vi "UHR-Fleezers Control (host) - 10.8.vi"() -> ()   [LabVIEW 2013] (continued)
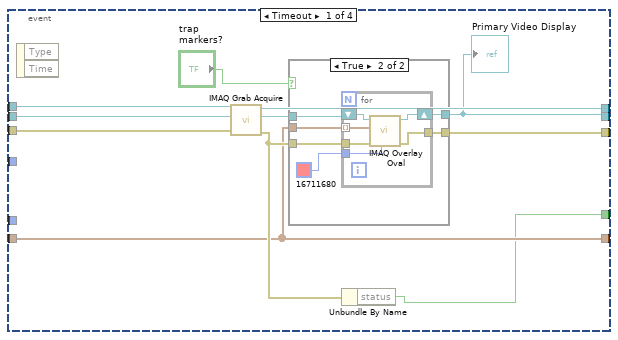
[diagram p2: hidden frame]
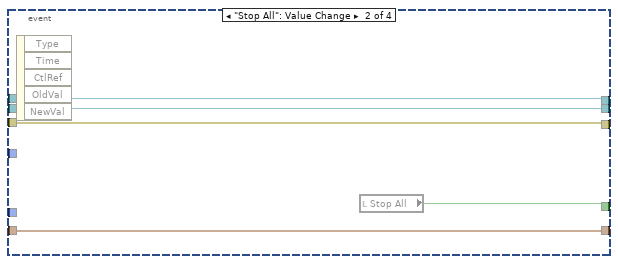
[diagram p4: hidden frame]
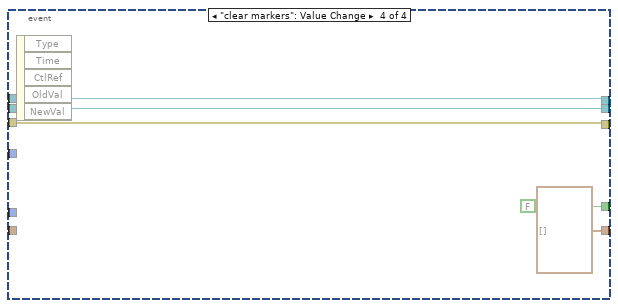
[diagram p6: hidden frame]
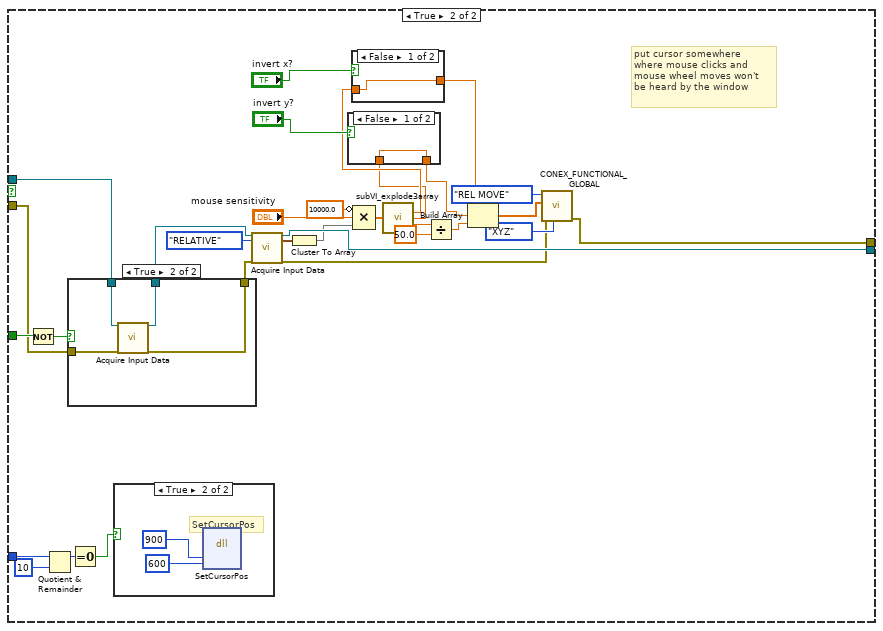
[diagram p9: hidden frame]
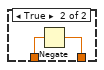
[diagram p12: hidden frame]
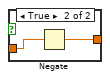
[diagram p13: hidden frame]
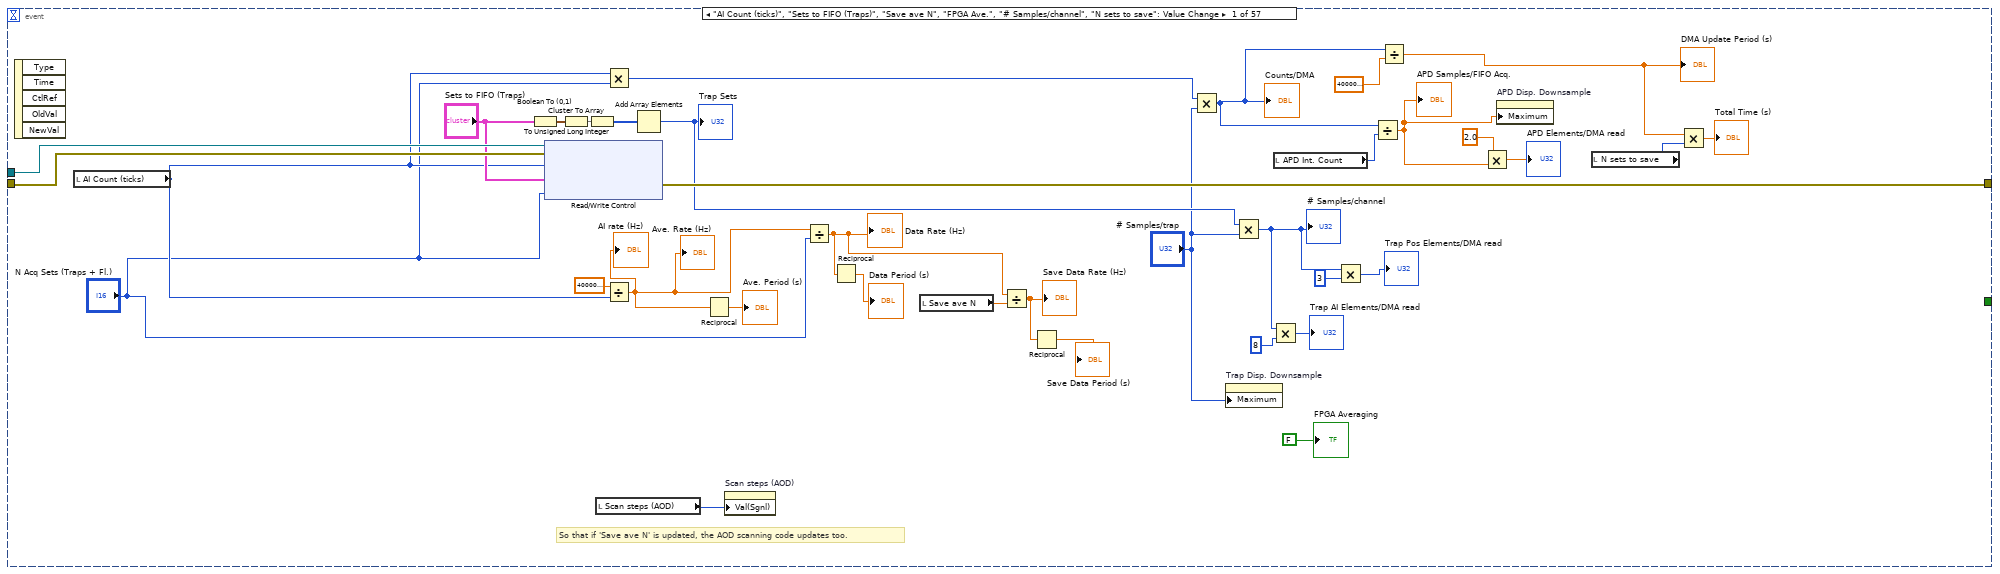
[diagram p14: hidden frame]
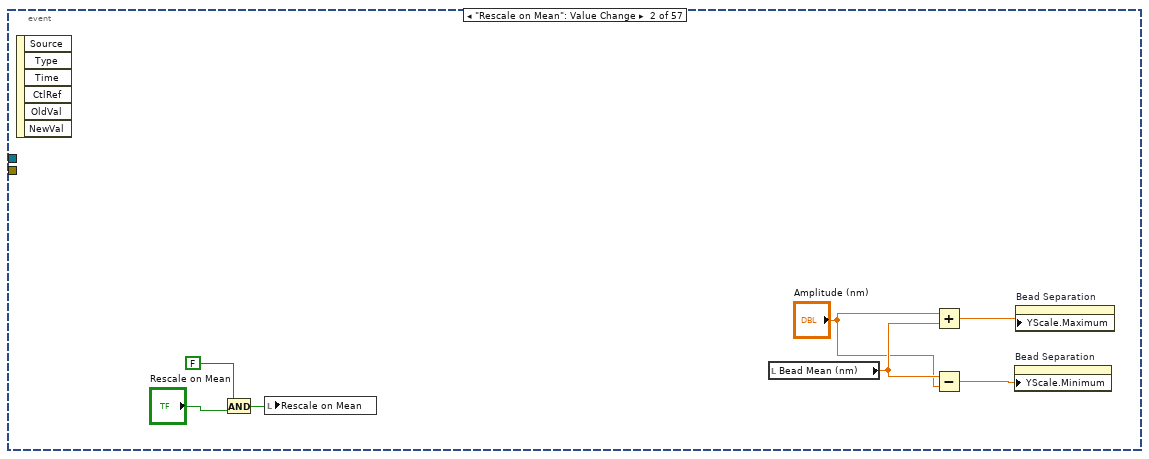
[diagram p15: hidden frame]
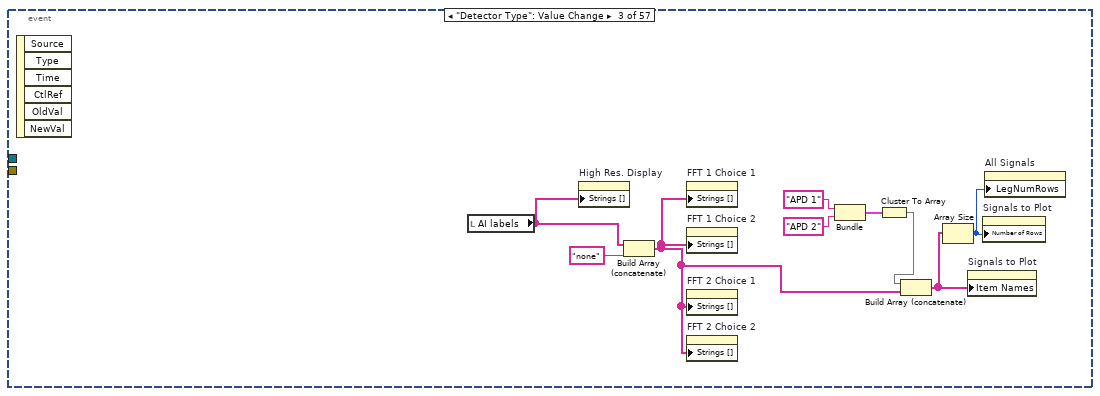
[diagram p16: hidden frame]
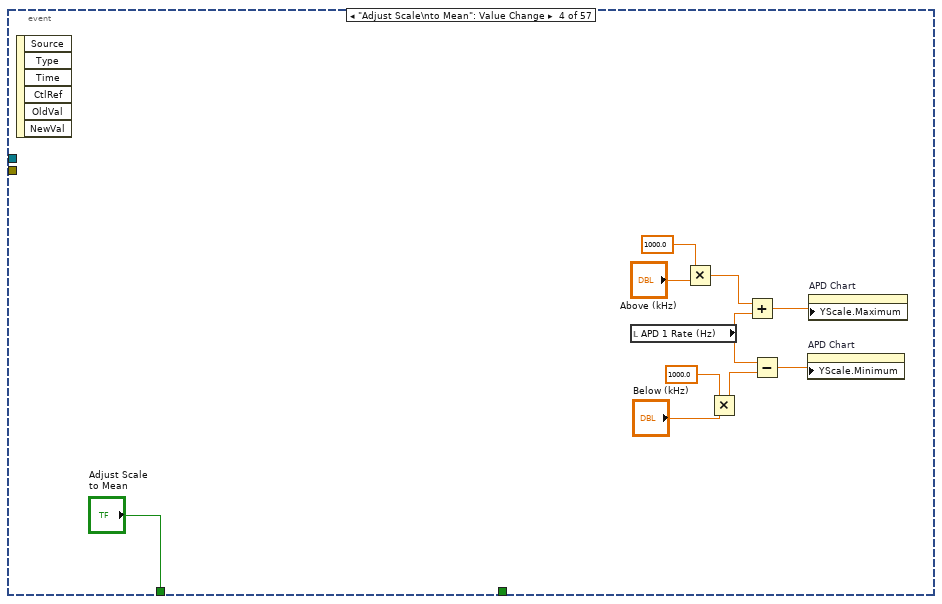
[diagram p17: hidden frame]
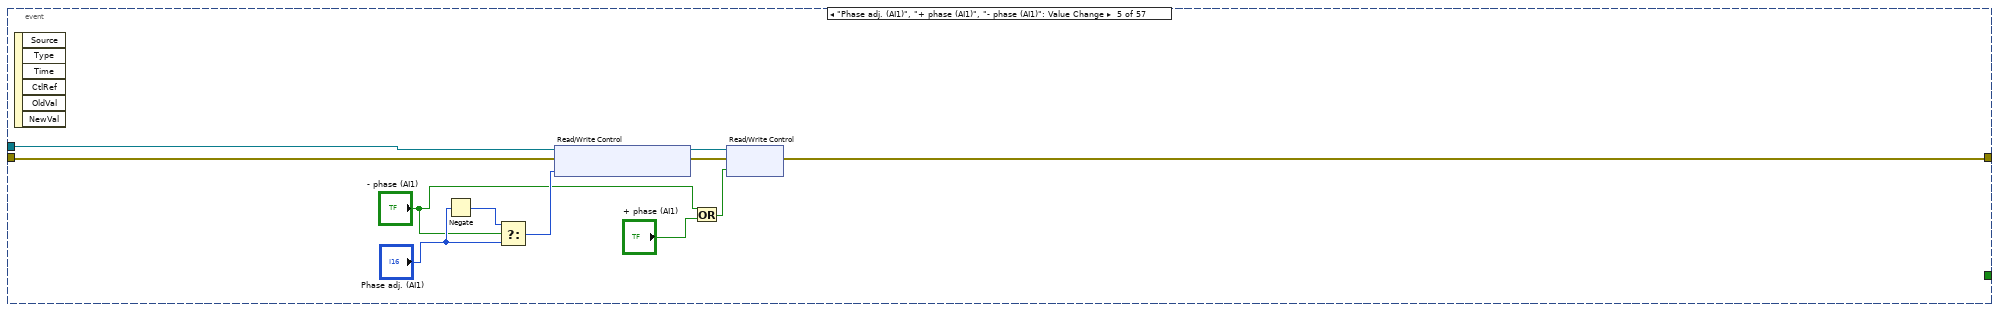
[diagram p18: hidden frame]
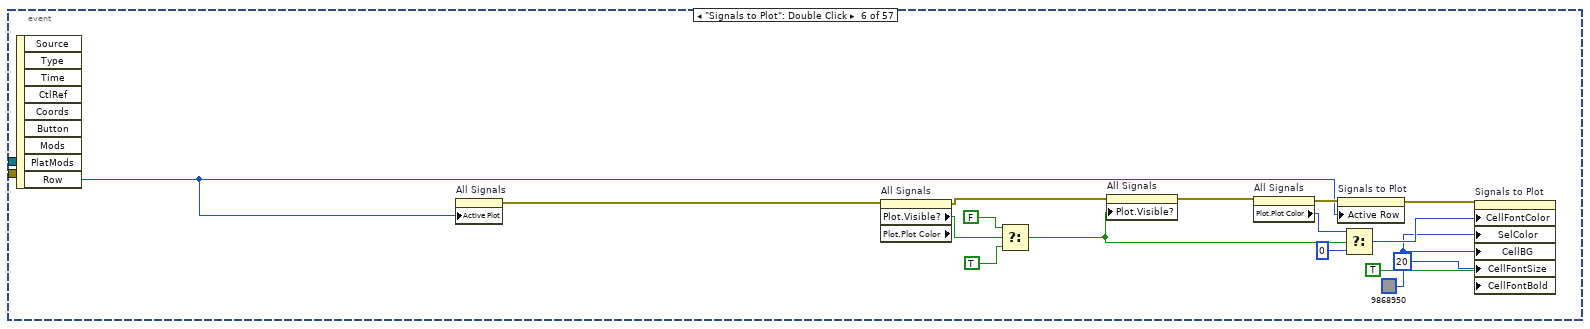
[diagram p19: hidden frame]
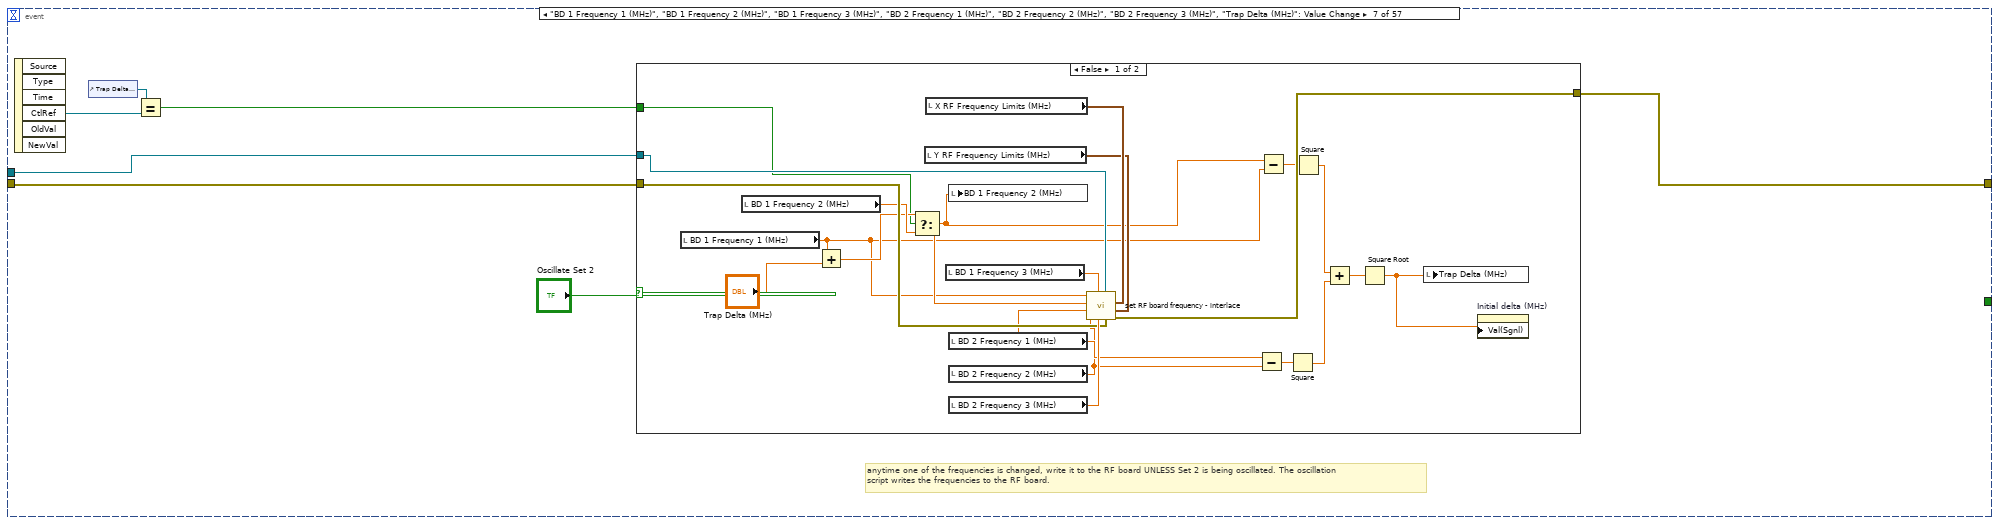
[diagram p20: hidden frame]
        n2049 = local read "Scan Range (V)\n(of steps)"() -> (w3461:dbl)
        n2050 = property on="Scan Range (V)\n(of steps)" class="DigNum (strict)"("Val(Sgnl)"=w3461) -> ()  [unwired: 2 in, 2 out]
      }
    }
    n2051 = node-c288() -> ()  [unwired: 2 out]
  }
  n2052 = node-c288(3 ("Processor")) -> (w73:T24)  [unwired: 3 out]
  n2053 = timed-loop "Mouse control: trap position (AOM deflection), set confocal spot from image" {
    tunnel: [w4497] -> w31
    tunnel: w16 -> [w4496]
    timing: w75 -> [_]
    timing-out: [_] -> w74
    stop <- w4497 stop-if-true
    n2054 = node-c288() -> ()  [unwired: 2 out]
    n2055 = event shown="[0] \"Pane\": Mouse Down" {
      selector: _ -> [_ _]
      dyn-events: _ -> [_ _]
      timeout: _ -> [_ _]
      tunnel: w4496 -> [w4500 _]
      event Mouse Down {
        n2056 = event-data() -> ("Time"=w4502:u32, "Coords"=w4501:T7, "Button"=w4503:u16)  [unwired: 6 out]
        n2057 = case shown="1" w4503 {
          tunnel: w4502 -> [_ _ w4606]
          tunnel: w4501 -> [_ w4540 w4604]
          tunnel: w4500 -> [_ _ w4602]
          frame 0, Default {
          }
          frame 1 {
            n2058 = property on="APD 2" class="ImageControl"() -> ("Displayed Image Position"=w4510:cluster{"Left":i32, "Top":i32})  [unwired: 2 in, 2 out]
            n2059 = property on="APD 1" class="ImageControl"() -> ("Displayed Image Position"=w4539:cluster{"Left":i32, "Top":i32})  [unwired: 2 in, 2 out]
            n2060 = property on="Detection Laser X" class="ImageControl"() -> ("Displayed Image Position"=w4536:cluster{"Left":i32, "Top":i32})  [unwired: 2 in, 2 out]
            n2061 = property on="Detection Laser Y" class="ImageControl"() -> ("Displayed Image Position"=w4535:cluster{"Left":i32, "Top":i32})  [unwired: 2 in, 2 out]
            n2062 = property on="APD 2" class="ImageControl"() -> ("Displayed Image Size"=w4509:cluster{"Width":u32, "Height":u32})  [unwired: 2 in, 2 out]
            n2063 = property on="APD 1" class="ImageControl"() -> ("Displayed Image Size"=w4537:cluster{"Width":u32, "Height":u32})  [unwired: 2 in, 2 out]
            n2064 = property on="Detection Laser X" class="ImageControl"() -> ("Displayed Image Size"=w4538:cluster{"Width":u32, "Height":u32})  [unwired: 2 in, 2 out]
            n2065 = property on="Detection Laser Y" class="ImageControl"() -> ("Displayed Image Size"=w4534:cluster{"Width":u32, "Height":u32})  [unwired: 2 in, 2 out]
            n2066 = Unbundle By Name(w4509) -> ("Width"=w4506:u32, "Height"=w4505:u32)
            n2067 = Unbundle By Name(w4510) -> ("Left"=w4508:i32, "Top"=w4507:i32)
            n2068 = Unbundle By Name(w4537) -> ("Width"=w4531:u32, "Height"=w4530:u32)
            n2069 = Unbundle By Name(w4538) -> ("Width"=w4527:u32, "Height"=w4526:u32)
            n2070 = Unbundle By Name(w4534) -> ("Width"=w4523:u32, "Height"=w4522:u32)
            n2071 = Unbundle By Name(w4539) -> ("Left"=w4533:i32, "Top"=w4532:i32)
            n2072 = Unbundle By Name(w4536) -> ("Left"=w4529:i32, "Top"=w4528:i32)
            n2073 = Unbundle By Name(w4535) -> ("Left"=w4525:i32, "Top"=w4524:i32)
            n2074 = Bundle("Left"=w4508, "Top"=w4507, "Width"=w4506, "Height"=w4505) -> (w4504:T52)  [unwired: 1 in]
            n2075 = Bundle("Left"=w4533, "Top"=w4532, "Width"=w4531, "Height"=w4530) -> (w4521:T52)  [unwired: 1 in]
            n2076 = Bundle("Left"=w4529, "Top"=w4528, "Width"=w4527, "Height"=w4526) -> (w4520:T52)  [unwired: 1 in]
            n2077 = Bundle("Left"=w4525, "Top"=w4524, "Width"=w4523, "Height"=w4522) -> (w4519:T52)  [unwired: 1 in]
            n2078 = Build Cluster Array(w4504, w4521, w4520, w4519) -> (w4518:T53)
            n2079 = for {
              tunnel: w4540 -> [w4551]
              tunnel: w4518 -> [w4552] mode=indexing
              shift-right: [w4549] -> w4516
              shift-left: TRUE -> [w4550]
              shift-right: [w4548] -> w4514
              shift-left: _ -> [w4544]
              shift-right: [w4547] -> w4513
              shift-left: _ -> [w4543]
              shift-right: [w4546] -> w4512
              shift-left: _ -> [w4542]
              shift-right: [w4545] -> w4511
              shift-left: _ -> [w4541]
              n2080 = case shown="True" w4550 {
                selector: w4550 -> [w4557 _]
                tunnel: w4552 -> [_ w4566]
                tunnel: w4551 -> [_ w4564]
                tunnel: [w4557 w4562] -> w4549
                tunnel: [w4556 w4561] -> w4548
                tunnel: [w4555 w4560] -> w4547
                tunnel: [w4554 w4559] -> w4546
                tunnel: [w4553 w4558] -> w4545
                tunnel: w4544 -> [w4556 _]
                tunnel: w4543 -> [w4555 _]
                tunnel: w4542 -> [w4554 _]
                tunnel: w4541 -> [w4553 _]
                frame False {
                }
                frame True {
                  n2081 = Unbundle(w4566) -> (w4565:T52)
                  n2082 = call "isclickinwindow.vi"("Image Param"=w4565, "Point32"=w4564) -> ("4 Y"=w4558:i32, "3 Height"=w4559:i32, "2 X"=w4560:i32, "1 Width"=w4561:i32, "In image?"=w4563:bool)  [unwired: 1 in]
                  n2083 = Not(x=w4563) -> (.not. x?=w4562:bool)
                }
              }
            }
            n2084 = Not(x=w4516) -> (.not. x?=w4515:bool)
            n2085 = case shown="True" w4515 {
              tunnel: w4513 -> [_ w4579]
              tunnel: w4511 -> [_ w4578]
              tunnel: w4514 -> [_ w4577]
              tunnel: w4512 -> [_ w4576]
              frame False {
              }
              frame True {
                w4572 = FALSE ("Get Point")
                n2086 = local read "Scan lines (y)"() -> (w4581:u64)
                n2087 = local read "Actual MCL Inc (V)"() -> (w4573:dbl)
                n2088 = local read "Scan steps (MCL)"() -> (w4580:u64)
                n2089 = Divide "Y Pix/step"(x=w4576, y=w4581) -> (x/y=w4588:dbl)
                n2090 = Divide "Y V/pix"(x=w4573, y=w4588) -> (x/y=w4587:dbl)
                n2091 = Divide "Y half step offset"(x=w4573, y=2.0) -> (x/y=w4589:dbl)
                n2092 = Divide "X pix/step"(x=w4577, y=w4580) -> (x/y=w4586:dbl)
                n2093 = Negate(x=w4589) -> (-x=w4590:dbl)
                n2094 = local read "Initial Y"() -> (w4596:dbl)
                n2095 = Multiply(x=w4578, y=w4587) -> (x*y=w4597:dbl)
                n2096 = Divide "X half step offset"(x=w4573, y=2.0) -> (x/y=w4583:dbl)
                n2097 = Divide "X V/pix"(x=w4573, y=w4586) -> (x/y=w4585:dbl)
                n2098 = Multiply(x=w4573, y=w4580) -> (x*y=w4592:dbl)
                n2099 = Compound Arithmetic op=ADD(w4590, w4597, w4596) -> (w4574:dbl)
                "Pointer Y (V)" <- w4574
                n2100 = Multiply(x=w4585, y=w4579) -> (x*y=w4594:dbl)
                n2101 = Negate(x=w4583) -> (-x=w4582:dbl)
                n2102 = local read "Initial X"() -> (w4595:dbl)
                n2103 = Negate(x=w4594) -> (-x=w4593:dbl)
                n2104 = Compound Arithmetic op=ADD(w4582, w4592, w4595, w4593) -> (w4575:dbl)
                "Pointer X (V)" <- w4575
                n2105 = Or(x="Set X Only", y="Set Confocal Spot (X-Y)") -> (x .or. y?=w4568:bool)
                n2106 = Or(x="Set Confocal Spot (X-Y)", y="Set Y Only") -> (x .or. y?=w4567:bool)
                n2107 = case shown="True" w4568 {
                  tunnel: w4575 -> [_ w4598]
                  frame False {
                  }
                  frame True {
                    n2108 = property on="AO2" class="Slide (strict)"("Val(Sgnl)"=w4598) -> ()  [unwired: 2 in, 2 out]
                  }
                }
                n2109 = case shown="True" w4567 {
                  tunnel: w4574 -> [_ w4599]
                  frame False {
                  }
                  frame True {
                    n2110 = property on="AO1" class="Slide (strict)"("Val(Sgnl)"=w4599) -> ()  [unwired: 2 in, 2 out]
                  }
                }
                n2111 = local write "Set Confocal Spot (X-Y)"(w4572) -> ()
                n2112 = local write "Set X Only"(w4572) -> ()
                n2113 = local write "Set Y Only"(w4572) -> ()
              }
            }
          }
          frame 3 {
            n2114 = local read "BD 2 Frequency 1 (MHz)"() -> (w4600:dbl)
            n2115 = local read "BD 1 Frequency 1 (MHz)"() -> (w4601:dbl)
            n2116 = local write "Manipulating Trap"(TRUE ("Manipulating Trap")) -> ()
            n2117 = local write "Coords"(T7 {"Horizontal"=0, "Vertical"=0} ("Coords")) -> ()
            n2118 = while {
              tunnel: w4606 -> [w4611]
              tunnel: w4604 -> [w4610]
              tunnel: w4602 -> [w4609]
              tunnel: w4601 -> [w4608]
              tunnel: w4600 -> [w4607]
              stop <- w4612 stop-if-true
              n2119 = event shown="[0] \"Pane\": Mouse Move" {
                selector: _ -> [_ _]
                dyn-events: _ -> [_ _]
                timeout: _ -> [_ _]
                tunnel: ["Force Manip Abort" w4676] -> w4612
                tunnel: w4611 -> [w4619 _]
                tunnel: w4610 -> [w4617 _]
                tunnel: w4609 -> [w4616 _]
                tunnel: w4608 -> [w4615 _]
                tunnel: w4607 -> [w4614 _]
                event Mouse Move {
                  n2120 = event-data() -> ("Time"=w4620:u32, "Coords"=w4621:T7)  [unwired: 3 out]
                  n2121 = Less?(x=w4620, y=w4619) -> (x < y?=w4618:bool)
                  n2122 = case "Makes sure old motion events prior to mouse click aren't used" shown="False" w4618 {
                    tunnel: w4621 -> [w4663 _]
                    tunnel: w4617 -> [w4664 _]
                    tunnel: w4616 -> [w4641 _]
                    tunnel: w4615 -> [w4637 _]
                    tunnel: w4614 -> [w4636 _]
                    frame False {
                      n2123 = Subtract(x=w4663, y=w4664) -> (x-y=w4662:T7)
                      "Coords" <- w4662
                      n2124 = local read "Y RF Frequency Limits (MHz)"() -> (w4622:T16)
                      n2125 = To Double Precision Float(number=w4662) -> (double precision float=w4661:cluster{"Horizontal":dbl, "Vertical":dbl})
                      n2126 = Multiply(x=cluster{"Horizontal":dbl, "Vertical":dbl} {"Horizontal"=-1.0, "Vertical"=1.0}, y="Manipulation Scaling") -> (x*y=w4657:cluster{"Horizontal":dbl, "Vertical":dbl})
                      n2127 = local read "X RF Frequency Limits (MHz)"() -> (w4623:T16)
                      n2128 = Multiply(x=w4661, y=w4657) -> (x*y=w4659:cluster{"Horizontal":dbl, "Vertical":dbl})
                      n2129 = Unbundle By Name(w4659) -> ("Horizontal"=w4654:dbl, "Vertical"=w4658:dbl)
                      n2130 = Unbundle By Name(w4622) -> ("Maximum"=w4625:dbl, "Minimum"=w4624:dbl)
                      n2131 = Boolean To (0,1)(Boolean="Manip. X?") -> (0, 1=w4652:i16)
                      n2132 = Boolean To (0,1)(Boolean="Manip. Y?") -> (0, 1=w4649:i16)
                      n2133 = local read "BD 1 Frequency 2 (MHz)"() -> (w4639:dbl)
                      n2134 = Multiply(x=w4658, y=w4649) -> (x*y=w4651:dbl)
                      n2135 = Multiply(x=w4652, y=w4654) -> (x*y=w4655:dbl)
                      n2136 = local read "BD 2 Frequency 2 (MHz)"() -> (w4638:dbl)
                      n2137 = Unbundle By Name(w4623) -> ("Maximum"=w4627:dbl, "Minimum"=w4626:dbl)
                      n2138 = Add(x=w4636, y=w4651) -> (x+y=w4629:dbl)
                      n2139 = Add(x=w4637, y=w4655) -> (x+y=w4631:dbl)
                      n2140 = In Range and Coerce(upper limit=w4627, x=w4631, lower limit=w4626) -> (coerced(x)=w4630:dbl)  [unwired: 1 out]
                      n2141 = In Range and Coerce(upper limit=w4625, x=w4629, lower limit=w4624) -> (coerced(x)=w4628:dbl)  [unwired: 1 out]
                      n2142 = Subtract(x=w4630, y=w4639) -> (x-y=w4648:dbl)
                      n2143 = Subtract(x=w4628, y=w4638) -> (x-y=w4647:dbl)
                      n2144 = Square(x=w4648) -> (x^2=w4646:dbl)
                      n2145 = Square(x=w4647) -> (x^2=w4645:dbl)
                      n2146 = Add(x=w4646, y=w4645) -> (x+y=w4644:dbl)
                      n2147 = Square Root(x=w4644) -> (sqrt(x)=w4640:dbl)
                      n2148 = In Range and Coerce(upper limit="Limit Max (MHz)", x=w4640, lower limit="Limit Min (MHz)") -> (In Range?=w4633:bool)  [unwired: 1 out]
                      n2149 = Not(x="Limits Enable") -> (.not. x?=w4632:bool)
                      n2150 = Or(x=w4633, y=w4632) -> (x .or. y?=w4634:bool)
                      n2151 = case shown="True" w4634 {
                        tunnel: w4641 -> [_ w4674]
                        tunnel: w4640 -> [_ w4665]
                        tunnel: w4630 -> [_ w4672]
                        tunnel: w4639 -> [_ w4671]
                        tunnel: w4628 -> [_ w4670]
                        tunnel: w4638 -> [_ w4669]
                        tunnel: w4623 -> [_ w4667]
                        tunnel: w4622 -> [_ w4666]
                        frame False {
                        }
                        frame True {
                          n2152 = local read "BD 1 Frequency 3 (MHz)"() -> (w4673:dbl)
                          n2153 = local read "BD 2 Frequency 3 (MHz)"() -> (w4668:dbl)
                          n2154 = local write "Trap Delta (MHz)"(w4665) -> ()
                          n2155 = property on="Initial delta (MHz)" class="DigNum (strict)"("Val(Sgnl)"=w4665) -> ()  [unwired: 2 in, 2 out]
                          n2156 = call "set RF board frequency - interlace.vi"("Board 2 Frequency Limits"=w4666, "Board 1 Frequency Limits"=w4667, "FPGA VI Reference In"=w4674, "Board 2 Frequency 3 (MHz)"=w4668, "Board 1 Frequency 3 (MHz)"=w4673, "Board 2 Frequency 2 (MHz)"=w4669, "Board 2 Frequency 1 (MHz)"=w4670, "Board 1 Frequency 2 (MHz)"=w4671, "Board 1 Frequency 1  (MHz)"=w4672) -> ()  [unwired: 1 in, 2 out]
                          n2157 = local write "BD 2 Frequency 1 (MHz)"(w4670) -> ()
                          n2158 = local write "BD 1 Frequency 1 (MHz)"(w4672) -> ()
                        }
                      }
                    }
                    frame True {
                    }
                  }
                }
                event Mouse Up {
                  n2159 = event-data() -> ("Button"=w4675:u16)  [unwired: 8 out]
                  n2160 = case shown="3" w4675 {
                    tunnel: [FALSE TRUE] -> w4676
                    frame 0, Default {
                    }
                    frame 3 {
                      n2161 = local write "Manipulating Trap"(FALSE ("Manipulating Trap")) -> ()
                    }
                  }
                }
              }
            }
          }
        }
      }
      event Mouse Move {
        n2162 = event-data() -> ()  [unwired: 6 out]
      }
    }
    n2163 = local read "Stop All"() -> (w4497:bool)
    n2164 = node-c288() -> ()  [unwired: 2 out]
  }
  n2165 = timed-loop "Oscillate AOD (debugging)" {
    tunnel: w16 -> [w4681]
    tunnel: [w4680] -> w33
    timing: w73 -> [_]
    timing-out: [_] -> w72
    stop <- w4680 stop-if-true
    n2166 = node-c288() -> ()  [unwired: 2 out]
    n2167 = event shown="[0] \"Oscillate Set 2\", \"Fish for Tether\": Value Change" {
      selector: _ -> [_ _ _]
      dyn-events: _ -> [_ _ _]
      timeout: _ -> [_ _ _]
      tunnel: w4681 -> [w4688 _ _]
      tunnel: [FALSE ("Stop All") _ w4956] -> w4680
      event "Oscillate Set 2", "Fish for Tether": Value Change {
        n2168 = event-data() -> ()  [unwired: 6 out]
        n2169 = local read "Oscillate Set 2"() -> (w4687:bool)
        n2170 = Or(x=w4687, y="Fish for Tether") -> (x .or. y?=w4685:bool)
        n2171 = case shown="True" w4685 {
          tunnel: w4688 -> [_ w4691]
          tunnel: "Fish for Tether" -> [_ w4690]
          frame False {
          }
          frame True {
            n2172 = case shown="True" w4690 {
              frame False {
              }
              frame True {
                n2173 = local write "Scan axis 2"(TRUE) -> ()
                n2174 = local write "Tether"(FALSE ("Tether")) -> ()
              }
            }
            n2175 = node-c288("Period") -> (w4693:T24)  [unwired: 3 out]
            n2176 = timed-loop "Oscillate AOD" {
              timing: w4693 -> [_]
              timing-out: [_] -> w4692
              tunnel: w4691 -> [w4703]
              tunnel: w4690 -> [w4702]
              i -> [w4705]
              stop <- w4701 stop-if-true
              n2177 = node-c288() -> (w4704:i64)  [unwired: 1 out]
              n2178 = flat-sequence {
                tunnel: w4705 -> [w4731]
                tunnel: w4704 -> [w4730]
                tunnel: w4703 -> [w4714]
                tunnel: w4702 -> [w4716]
                tunnel: [w4716] -> w4700
                tunnel: [w4715] -> w4699
                tunnel: [w4713] -> w4698
                tunnel: [w4710] -> w4696
                tunnel: w4700 -> [w4767]
                tunnel: w4699 -> [w4765]
                tunnel: w4698 -> [w4764]
                tunnel: [w4763] -> w4697
                tunnel: w4696 -> [w4762]
                tunnel: [w4831] -> w4701
                tunnel: w4697 -> [w4829]
                frame #0 {
                  n2179 = Divide(x=w4730, y=i64 1000) -> (x/y=w4725:dbl)
                  n2180 = Multiply(x=w4725, y=w4731) -> (x*y=w4727:dbl)
                  n2181 = Multiply(x="Osc. freq. (Hz)", y=6.283185307179586) -> (x*y=w4728:dbl)
                  n2182 = Multiply(x=w4728, y=w4727) -> (x*y=w4712:dbl)
                  n2183 = local read "BD 1 Frequency 2 (MHz)"() -> (w4709:dbl)
                  n2184 = local read "BD 1 Frequency 1 (MHz)"() -> (w4706:dbl)
                  n2185 = case shown="True" w4716 {
                    tunnel: w4712 -> [w4737 w4744]
                    tunnel: w4709 -> [_ w4754]
                    tunnel: [w4734 w4738] -> w4717
                    tunnel: [FALSE w4747] -> w4713
                    tunnel: [0.0 w4740] -> w4710
                    tunnel: w4706 -> [_ w4739]
                    frame False {
                      n2186 = Sine(x=w4737) -> (sin(x)=w4735:dbl)
                      n2187 = Multiply(x=w4735, y="Osc. amp. (MHz)") -> (x*y=w4734:dbl)
                    }
                    frame True {
                      n2188 = Cosine(x=w4744) -> (cos(x)=w4757:dbl)
                      n2189 = Subtract(x=w4754, y=w4739) -> (x-y=w4753:dbl)
                      n2190 = Decrement(x=w4757) -> (x-1=w4756:dbl)
                      n2191 = Subtract(x=w4753, y="Closest Delta (MHz)") -> (x-y=w4750:dbl)
                      n2192 = Divide(x=w4756, y=2.0) -> (x/y=w4751:dbl)
                      n2193 = Multiply(x=w4751, y=w4750) -> (x*y=w4738:dbl)
                      n2194 = local read "Vec Mean of T1 T2"() -> (w4746:dbl[])
                      n2195 = Greater?(x=w4746, y="Stop F (pN)") -> (0:w4748:bool[])
                      n2196 = Or Array Elements(Boolean array=w4748) -> (logical OR=w4747:bool)
                      n2197 = Divide(x=w4744, y=6.283185307179586) -> (x/y=w4743:dbl)
                      n2198 = Round Toward +Infinity(x=w4743) -> (ceil(x): smallest int >= x=w4740:dbl)
                      "Attempts" <- w4740
                      n2199 = Greater?(x=w4740, y="Attempt Limit") -> (0:w4742:bool)
                      n2200 = case shown="True" w4742 {
                        frame False {
                        }
                        frame True {
                          n2201 = local write "Fish for Tether"(FALSE ("Fish for Tether")) -> ()
                          n2202 = call <vilib>:"Beep.vi"() -> ()  [unwired: 3 in, 9 out]
                          n2203 = local read "Messages"() -> (w4759:string)
                          n2204 = call "Update messages.vi"("Message to add"="Tether fishing timeout." ("Messages"), "Old message string"=w4759) -> ("New message string"=→"Messages":string)
                        }
                      }
                    }
                  }
                  n2205 = local read "Y RF Frequency Limits (MHz)"() -> (w4718:T16)
                  n2206 = local read "X RF Frequency Limits (MHz)"() -> (w4719:T16)
                  n2207 = local read "BD 1 Frequency 3 (MHz)"() -> (w4724:dbl)
                  n2208 = local read "BD 2 Frequency 2 (MHz)"() -> (w4708:dbl)
                  n2209 = Select(t=w4709, s="Scan axis 2", f=w4708) -> (s? t:f=w4720:dbl)
                  n2210 = Add(x=w4717, y=w4720) -> (x+y=w4715:dbl)
                  n2211 = Select(t=w4715, s="Scan axis 2", f=w4709) -> (s? t:f=w4707:dbl)
                  n2212 = Select(t=w4708, s="Scan axis 2", f=w4715) -> (s? t:f=w4722:dbl)
                  n2213 = local read "BD 2 Frequency 3 (MHz)"() -> (w4723:dbl)
                  n2214 = call "set RF board frequency - interlace.vi"("Board 2 Frequency Limits"=w4718, "Board 1 Frequency Limits"=w4719, "FPGA VI Reference In"=w4714, "Board 2 Frequency 3 (MHz)"=w4723, "Board 1 Frequency 3 (MHz)"=w4724, "Board 2 Frequency 2 (MHz)"=w4708, "Board 2 Frequency 1 (MHz)"=w4722, "Board 1 Frequency 2 (MHz)"=w4707, "Board 1 Frequency 1  (MHz)"=w4706) -> ()  [unwired: 1 in, 2 out]
                }
                frame #1 {
                  n2215 = And(x=w4767, y=w4764) -> (x .and. y?=w4766:bool)
                  n2216 = case "Only if were fishing and now formed tether" shown="True" w4766 {
                    tunnel: w4765 -> [w4769 w4781]
                    tunnel: [w4768 w4780] -> w4763
                    tunnel: w4762 -> [_ w4776]
                    frame False {
                      n2217 = local read "Fish for Tether"() -> (w4768:bool)
                      n2218 = case shown="True" w4768 {
                        tunnel: w4769 -> [_ _]
                        frame False {
                        }
                        frame True {
                        }
                      }
                    }
                    frame True {
                      w4780 = FALSE ("Fish for Tether")
                      n2219 = call <vilib>:"Beep.vi"() -> ()  [unwired: 3 in, 9 out]
                      n2220 = Number To Decimal String(number=w4776, width (-)=i16 1) -> (decimal integer string=w4774:string)
                      n2221 = case shown="\"2\", \"3\", \"4\", \"5\", \"6\"" "Then..." {
                        selector: "Then..." -> [_ w4784]
                        tunnel: w4781 -> [w4783 _]
                        frame "1", Default {
                          # "do nothing"
                          n2222 = property on="BD 1 Frequency 1 (MHz)" class="DigNum (strict)"("Val(Sgnl)"=w4783) -> ()  [unwired: 2 in, 2 out]
                        }
                        frame "2", "3", "4", "5", "6" {
                          n2223 = flat-sequence {
                            tunnel: w4784 -> [w4786]
                            frame #0 {
                              n2224 = property on="Trap Delta (MHz)" class="DigNum (strict)"("Val(Sgnl)"="Move to Delta 1 (MHz)") -> ()  [unwired: 2 in, 2 out]
                            }
                            frame #1 {
                              n2225 = case shown="\"5\", \"6\"" w4786 {
                                selector: w4786 -> [w4789 w4799 _]
                                frame "3", "4" {
                                n2226 = flat-sequence {
                                tunnel: w4789 -> [w4790]
                                tunnel: [w4790] -> w4787
                                tunnel: [w4792] -> w4788
                                tunnel: w4787 -> [w4792]
                                tunnel: w4788 -> [w4796]
                                frame #0 {
                                n2227 = property on="Green Laser ON/Interlacing" class="Bool (strict)"("Val(Sgnl)"=TRUE ("Value (Signaling)")) -> ()  [unwired: 2 in, 2 out]
                                }
                                frame #1 {
                                n2228 = Multiply(x="Wait Before Save (s)", y=u32 1000 ("x")) -> (x*y=w4794:u32)
                                n2229 = Wait (ms)(milliseconds to wait=w4794) -> ()  [unwired: 1 out]
                                }
                                frame #2 {
                                n2230 = property on="Start Saving" class="Bool (strict)"("Value"=TRUE ("Start Saving")) -> ()  [unwired: 2 in, 2 out]
                                n2231 = case shown="\"4\"" w4796 {
                                frame Default {
                                }
                                frame "4" {
                                n2232 = property on="Fl. Triggered..." class="Bool (strict)"("Val(Sgnl)"=TRUE ("Value (Signaling)")) -> ()  [unwired: 2 in, 2 out]
                                }
                                }
                                }
                                }
                                }
                                frame "5", "6" {
                                n2233 = stacked-sequence {
                                tunnel: w4799 -> [_ _ _ _ _ _ _ _ w4816 _ _]
                                frame #0 {
                                n2234 = Replace Array Subset(array=u32[] [0] ("Index Values"), new element="Raster Set Upon Tether", index=0) -> (w4800:u32[])
                                n2235 = property on="Saved AOD Raster Scan Parameter Sets" class="Arr (strict)"("Index Values"=w4800) -> ()  [unwired: 2 in, 2 out]
                                }
                                frame #1 {
                                n2236 = Wait (ms)(milliseconds to wait=u32 500) -> ()  [unwired: 1 out]
                                }
                                frame #2 {
                                n2237 = property on="Load parameters" class="Bool (strict)"("Val(Sgnl)"=TRUE ("Value (Signaling)")) -> ()  [unwired: 2 in, 2 out]
                                }
                                frame #3 {
                                n2238 = Wait (ms)(milliseconds to wait=u32 500) -> ()  [unwired: 1 out]
                                }
                                frame #4 {
                                n2239 = property on="Trap Raster Scan" class="Bool (strict)"("Val(Sgnl)"=TRUE ("Value (Signaling)")) -> ()  [unwired: 2 in, 2 out]
                                }
                                frame #5 {
                                n2240 = Wait (ms)(milliseconds to wait=u32 2000) -> ()  [unwired: 1 out]
                                }
                                frame #6 {
                                n2241 = while {
                                stop <- w4811 stop-if-true
                                n2242 = local read "Raster Scanning..."() -> (w4810:bool)
                                n2243 = local read "Saving..."() -> (w4813:bool)
                                n2244 = Wait (ms)(milliseconds to wait=u32 100) -> ()  [unwired: 1 out]
                                n2245 = Not(x=w4813) -> (.not. x?=w4812:bool)
                                n2246 = Not(x=w4810) -> (.not. x?=w4809:bool)
                                n2247 = And(x=w4812, y=w4809) -> (x .and. y?=w4811:bool)
                                }
                                }
                                frame #7 {
                                n2248 = property on="Trap Delta (MHz)" class="DigNum (strict)"("Val(Sgnl)"="Move to Delta 2 (MHz)") -> ()  [unwired: 2 in, 2 out]
                                }
                                frame #8 {
                                n2249 = local read "Tether"() -> (w4817:bool)
                                n2250 = case shown="True" w4817 {
                                tunnel: w4816 -> [_ w4818]
                                frame False {
                                }
                                frame True {
                                n2251 = flat-sequence {
                                tunnel: w4818 -> [w4820]
                                frame #0 {
                                n2252 = Wait (ms)(milliseconds to wait=u32 500) -> ()  [unwired: 1 out]
                                }
                                frame #1 {
                                n2253 = case shown="\"6\"" w4820 {
                                frame Default {
                                }
                                frame "6" {
                                n2254 = property on="Green Laser ON/Interlacing" class="Bool (strict)"("Val(Sgnl)"=TRUE ("Green Laser ON/Interlacing")) -> ()  [unwired: 2 in, 2 out]
                                }
                                }
                                }
                                frame #2 {
                                n2255 = Wait (ms)(milliseconds to wait=u32 500) -> ()  [unwired: 1 out]
                                }
                                frame #3 {
                                n2256 = local write "Start Saving"("Save at end (5, 6)") -> ()
                                }
                                }
                                }
                                }
                                }
                                frame #9 {
                                n2257 = local read "Bead Sep. Int. Time (s)"() -> (w4826:dbl)
                                n2258 = Multiply(x=w4826, y=1000.0) -> (x*y=w4825:dbl)
                                n2259 = Wait (ms)(milliseconds to wait=w4825) -> ()  [unwired: 1 out]
                                }
                                frame #10 {
                                n2260 = property on="Rescale on Mean" class="Bool (strict)"("Val(Sgnl)"=TRUE ("Value (Signaling)")) -> ()  [unwired: 2 in, 2 out]
                                }
                                }
                                }
                                frame "2", Default {
                                }
                              }
                            }
                          }
                        }
                      }
                      n2261 = Concatenate Strings("Formed tether in ", w4774, " attempt(s)." ("string")) -> (w4771:string)
                      n2262 = local read "Messages"() -> (w4778:string)
                      n2263 = local write "Fish for Tether"(w4780) -> ()
                      n2264 = call "Update messages.vi"("Message to add"=w4771, "Old message string"=w4778) -> ("New message string"=w4777:string)
                      n2265 = local write "Messages"(w4777) -> ()
                      n2266 = Get Date/Time In Seconds() -> (seconds since 1Jan1904=→"Time tether formed":timestamp)
                      "Tether" <- "Tether Alarm?"
                    }
                  }
                }
                frame #2 {
                  n2267 = local read "Oscillate Set 2"() -> (w4830:bool)
                  n2268 = local read "Stop All"() -> (w4832:bool)
                  n2269 = Not Or(1:w4829, 2:w4830) -> (0:w4828:bool)
                  n2270 = Compound Arithmetic op=OR(w4832, w4828) -> (w4831:bool)
                }
              }
              n2271 = node-c288() -> ()  [unwired: 2 out]
            }
            n2272 = node-c288(w4692) -> ()  [unwired: 1 out]
          }
        }
      }
      event "Fl. Triggered...": Value Change {
        n2273 = event-data() -> ()  [unwired: 7 out]
        n2274 = case shown="True" "Fl. Triggered..." {
          frame False {
          }
          frame True {
            n2275 = node-c288() -> (w4844:T24)  [unwired: 4 out]
            n2276 = timed-loop {
              timing: w4844 -> [_]
              timing-out: [_] -> w4843
              tunnel: "Action" -> [w4848]
              shift-right: [w4845] -> _
              shift-left: u8 255 -> [w4847]
              stop <- w4849 stop-if-true
              n2277 = node-c288() -> ()  [unwired: 2 out]
              n2278 = flat-sequence {
                tunnel: w4848 -> [w4861]
                tunnel: w4847 -> [w4858]
                tunnel: [w4857] -> w4846
                tunnel: [w4947] -> w4849
                tunnel: w4846 -> [w4946]
                tunnel: [w4946] -> w4845
                frame #0 {
                  n2279 = local read "Delta Fl. 2"() -> (w4852:dbl)
                  n2280 = local read "Delta Fl. 1"() -> (w4853:dbl)
                  n2281 = Select(t=w4853, s="APD to Watch", f=w4852) -> (s? t:f=w4851:dbl)
                  n2282 = Multiply(x="Fl. Delta Thresh. (kHz)", y=1000.0) -> (x*y=w4860:dbl)
                  n2283 = Greater?(x=w4851, y=w4860) -> (0:w4855:bool)
                  n2284 = Or(x="Force Yank", y=w4855) -> (x .or. y?=w4856:bool)
                  n2285 = case shown="True" w4856 {
                    tunnel: w4861 -> [_ w4871]
                    tunnel: w4858 -> [w4863 w4867]
                    tunnel: [w4863 w4864] -> w4857
                    frame False {
                    }
                    frame True {
                      n2286 = flat-sequence {
                        tunnel: w4868 -> [w4877]
                        tunnel: [w4877] -> w4872
                        tunnel: w4871 -> [w4876]
                        tunnel: [w4876] -> w4870
                        tunnel: [w4875] -> w4869
                        tunnel: w4867 -> [w4874]
                        tunnel: [w4873] -> w4866
                        tunnel: w4872 -> [w4902]
                        tunnel: w4870 -> [w4901]
                        tunnel: w4869 -> [w4900]
                        tunnel: w4866 -> [w4899]
                        tunnel: [w4899] -> w4865
                        tunnel: w4865 -> [w4944]
                        tunnel: [w4944] -> w4864
                        frame #0 {
                          n2287 = call <vilib>:"Beep.vi"() -> ()  [unwired: 3 in, 9 out]
                          n2288 = local write "Waiting"(FALSE ("Waiting")) -> ()
                          n2289 = Increment(x=w4874) -> (x+1=w4873:u8)
                          n2290 = case shown="\"Yank\"" w4876 {
                            tunnel: w4873 -> [_ _ w4883]
                            frame "Image" {
                              n2291 = property on="Confocal Image" class="Bool (strict)"("Val(Sgnl)"=TRUE ("Value (Signaling)")) -> ()  [unwired: 2 in, 2 out]
                            }
                            frame "Alarm", Default {
                            }
                            frame "Yank" {
                              n2292 = flat-sequence {
                                tunnel: w4883 -> [w4886]
                                tunnel: [w4885] -> w4882
                                tunnel: ["N Array El"] -> w4881
                                tunnel: w4882 -> [w4896]
                                tunnel: w4881 -> [w4892]
                                frame #0 {
                                n2293 = Multiply(x="Yank Delay (s)", y=1000.0) -> (x*y=w4889:dbl)
                                n2294 = Quotient & Remainder(x=w4886, y="N Array El") -> (x-y*floor(x/y)=w4885:u8)  [unwired: 1 out]
                                n2295 = Wait (ms)(milliseconds to wait=w4889) -> ()  [unwired: 1 out]
                                }
                                frame #1 {
                                n2296 = Random Number (0-1)() -> (number: 0 to 1=w4893:dbl)
                                n2297 = Multiply(x=w4892, y=w4893) -> (x*y=w4891:dbl)
                                n2298 = Round Toward -Infinity(1:w4891) -> (0:w4890:dbl)
                                n2299 = Select(t=w4890, s="Random Choice", f=w4896) -> (s? t:f=w4894:dbl)
                                n2300 = Index Array(array="Yank to Delta Array (MHz)", index=w4894) -> (element=w4897:dbl)
                                n2301 = property on="Trap Delta (MHz)" class="DigNum (strict)"("Val(Sgnl)"=w4897) -> ()  [unwired: 2 in, 2 out]
                                }
                              }
                            }
                          }
                          n2302 = local read "Time (s)"() -> (w4875:dbl)
                          "Fl. High" <- TRUE ("Yanking")
                        }
                        frame #1 {
                          n2303 = node-c288() -> (w4904:T24)  [unwired: 4 out]
                          n2304 = timed-loop {
                            timing: w4904 -> [_]
                            timing-out: [_] -> w4903
                            tunnel: w4902 -> [w4920]
                            tunnel: w4901 -> [w4918]
                            tunnel: w4900 -> [w4917]
                            stop <- w4919 stop-if-true
                            n2305 = node-c288() -> ()  [unwired: 2 out]
                            n2306 = local read "Fl. Delta Thresh. (kHz)"() -> (w4912:dbl)
                            n2307 = local read "Fl. Triggered..."() -> (w4921:bool)
                            n2308 = local read "Delta Fl. 1"() -> (w4908:dbl)
                            n2309 = local read "Delta Fl. 2"() -> (w4906:dbl)
                            n2310 = local read "Stop All"() -> (w4915:bool)
                            n2311 = local read "APD to Watch"() -> (w4907:bool)
                            n2312 = Select(t=w4908, s=w4907, f=w4906) -> (s? t:f=w4905:dbl)
                            n2313 = Not(x=w4921) -> (.not. x?=w4916:bool)
                            n2314 = Multiply(x=w4912, y=1000.0) -> (x*y=w4911:dbl)
                            n2315 = Negate(x=w4911) -> (-x=w4910:dbl)
                            n2316 = Less?(x=w4905, y=w4910) -> (x < y?=w4914:bool)
                            n2317 = Compound Arithmetic op=OR(w4914, w4915, w4916, "Force Reset") -> (w4919:bool)
                            n2318 = case shown="True" w4919 {
                              tunnel: w4920 -> [_ w4932]
                              tunnel: w4918 -> [_ w4931]
                              tunnel: w4917 -> [_ w4929]
                              frame False {
                              }
                              frame True {
                                n2319 = case shown="\"Yank\"" w4931 {
                                tunnel: w4932 -> [_ w4933]
                                frame "Image", Default {
                                }
                                frame "Yank" {
                                n2320 = flat-sequence {
                                tunnel: [w4938] -> w4934
                                tunnel: w4933 -> [w4938]
                                tunnel: w4934 -> [w4939]
                                frame #0 {
                                n2321 = local read "Yank Delay (s)"() -> (w4937:dbl)
                                n2322 = Multiply(x=w4937, y=1000.0) -> (x*y=w4935:dbl)
                                n2323 = Wait (ms)(milliseconds to wait=w4935) -> ()  [unwired: 1 out]
                                }
                                frame #1 {
                                n2324 = property on="Trap Delta (MHz)" class="DigNum (strict)"("Val(Sgnl)"=w4939) -> ()  [unwired: 2 in, 2 out]
                                }
                                }
                                }
                                }
                                n2325 = local read "Time (s)"() -> (w4930:dbl)
                                n2326 = Subtract(x=w4930, y=w4929) -> (x-y=w4926:dbl)
                                "Duration (s)" <- w4926
                                n2327 = Number To Decimal String(number=w4926, width (-)=i16 0) -> (decimal integer string=w4924:string)
                                n2328 = Concatenate Strings(w4924, " s fluorescence event." ("string")) -> (w4922:string)
                                n2329 = local read "Messages"() -> (w4928:string)
                                n2330 = call "Update messages.vi"("Message to add"=w4922, "Old message string"=w4928) -> ("New message string"=w4927:string)
                                n2331 = call <vilib>:"Beep.vi"() -> ()  [unwired: 3 in, 9 out]
                                n2332 = local write "Messages"(w4927) -> ()
                              }
                            }
                            n2333 = node-c288() -> ()  [unwired: 2 out]
                          }
                          n2334 = node-c288(w4903) -> ()  [unwired: 1 out]
                        }
                        frame #2 {
                          n2335 = local write "Fl. High"(FALSE ("Yanking")) -> ()
                        }
                      }
                      n2336 = local read "Trap Delta (MHz)"() -> (w4868:dbl)
                    }
                  }
                }
                frame #1 {
                  n2337 = local read "Stop All"() -> (w4950:bool)
                  n2338 = local read "Fl. Triggered..."() -> (w4948:bool)
                  n2339 = Not(x=w4948) -> (.not. x?=w4949:bool)
                  n2340 = Or(x=w4949, y=w4950) -> (x .or. y?=w4947:bool)
                  n2341 = Not(x=w4947) -> (.not. x?=→"Waiting":bool)
                }
              }
              n2342 = node-c288() -> ()  [unwired: 2 out]
            }
            n2343 = node-c288(w4843) -> ()  [unwired: 1 out]
          }
        }
      }
      event "Stop All": Value Change {
        n2344 = event-data() -> ()  [unwired: 7 out]
        n2345 = local read "Stop All"() -> (w4956:bool)
      }
    }
    n2346 = node-c288() -> ()  [unwired: 2 out]
  }
  n2347 = node-c288(w3) -> ()  [unwired: 1 out]
  n2348 = call-poly <vilib>:"Close Input Device.vi"("device ID"=w21) -> ()  [unwired: 9 in, 1 out]
  n2349 = node-c288(w6) -> ()  [unwired: 1 out]
  n2350 = node-c288(w67) -> ()  [unwired: 1 out]
  n2351 = node-c288(w74) -> ()  [unwired: 1 out]
  n2352 = node-c288(w72) -> ()  [unwired: 1 out]
  n2353 = node-c288(w162) -> ()  [unwired: 1 out]
  n2354 = flat-sequence {
    tunnel: w30 -> [w4961]
    tunnel: [w4960] -> w36
    tunnel: [w4957] -> w35
    tunnel: w34 -> [_]
    tunnel: w33 -> [_]
    tunnel: w32 -> [_]
    tunnel: w31 -> [_]
    tunnel: w29 -> [w4958]
    tunnel: w36 -> [w5023]
    tunnel: w35 -> [w5022]
    frame #0 {
      w4959 = FALSE ("APD to FIFO")
      n2355 = xnode "Read/Write Control"("FPGA VI Reference In"=w4961, "error in"=w4958, "APD to FIFO"=w4959, "AI to FIFO"=w4959) -> ("FPGA VI Reference Out"=w4960:T19, "error out"=w4957:errorcluster)
    }
    frame #1 {
      n2356 = xnode "Invoke Method"("FPGA VI Reference In"=w5023, "error in"=w5022) -> ("FPGA VI Reference Out"=w5021:T19)  [unwired: 1 out]
      n2357 = xnode "Close FPGA VI Reference"("FPGA VI Reference In"=w5021) -> ()  [unwired: 1 in, 1 out]
    }
  }
